vi "ALTS-2015 OPC Read Engine.vi"(8 "error in (no error)":errorcluster, 11 "Delay (ms)":u32=100) -> (0 "error out":errorcluster)   [LabVIEW 2013]
doc: "Copyright © 2005, Soliton Technologies.\nAll rights reserved."
uses:
  Controls/ALTS-2015 OPC Engine Main Options.ctl
  Controls/ALTS-2015 OPC Read Registers.ctl
  Controls/ALTS-2015 OPC Read Global Options.ctl
  Controls/ALTS-2015 OPC Global Options.ctl
  Controls/ALTS-2015 OPC Global Elements.ctl
  Globals/ALTS-2015 OPC Engine Globals.vi
  Controls/ALTS-2015 Safety Logic Cases.ctl
panel:
  in  "OPC Read Registers":T1=enum."Start_Test"
  out "Running Case":T2
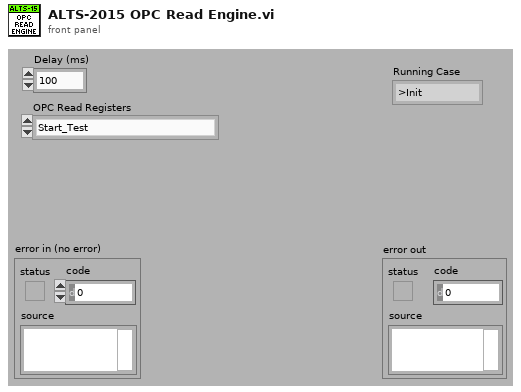
[diagram p1: front panel]
types:
  T1 = typedef "ALTS-2015 OPC Read Registers.ctl" = enum16{"Robot_Available", "Start_Test", "Stop_Test", "Scan_Trigger", "Station_No_Start_Stop_Test"}
  T2 = typedef "ALTS-2015 OPC Engine Main Options.ctl" = enum16{">Init", ">Safe Mode", ">Poll", ">Error", ">Exit", ">Write", ">Read", ">Restart"}
  T3 = typedef "ALTS-2015 OPC Global Options.ctl" = enum16{"Init", "Write 1", "Read 1", "Write Array", "Read Array", "Clear"}
  T4 = typedef "ALTS-2015 OPC Read Global Options.ctl" = enum16{"Init", "Write Value", "Write Array", "Read Value", "Read Array", "Read All"}
  T5 = cluster{"Channel Order":i32[], "Connection ids":refnum<k13>[]}
  T6 = enum16{"Read", "Write", "ReadWrite", "BufferedRead", "BufferedReadWrite"}
  T7 = typedef "ALTS-2015 OPC Global Elements.ctl" = enum16{"OPC - R Error", "OPC - W Error", "OPC - R Restart", "OPC - W Restart", "OPC - R Running", "OPC - W Running"}
  T8 = typedef "ALTS-2015 Safety Logic Cases.ctl" = enum16{"Read S/W EStop", "Read H/W EStop", "Write S/W EStop", "Write H/W EStop", "Read S/W & H/W EStop"}
  T9 = typedef "ALTS-2015 INI Configuration Cluster.ctl" = cluster{"Application":cluster{"Rerun Count":i32, "Workorder No":string}, "Station Details":cluster{"Sensor Name 1":string, "Sensor Name 2":string, "Sensor Name 3":string, "Sensor Name 4":string, "Station1 Enable":bool, "Station2 Enable":bool, "Station3 Enable":bool, "Station4 Enable":bool}, "Database":cluster{"Database Connection Link":path, "Result Procedure":string, "User":string, "Password":string, "Prompt":bool, "Station 1 LT Result DB DSN Path":path, "Station 2 LT Result DB DSN Path":path, "Station 3 LT Result DB DSN Path":path, "Station 4 LT Result DB DSN Path":path, "AirLeakTestResult Procedure":string, "Serial Details Procedure":string}, "Simulation":cluster{"Simulate DAQ Hardware":bool, "Simulate Result DB Write":bool, "Simulate Scanner":bool, "Simulate OPC":bool, "Simulate Serial Details DB":bool, "Simulate Result DB":bool, "Simulate Scanner DB Path":path, "Simulate Serial Details DB Path":path, "Simulate Result DB Path":path}, "Barcode Scanner1":cluster{"Scanner IP":string, "Scanner Port":u16, "#Bytes to Read":i32}, "Barcode Scanner2":cluster{"Enabled?":bool, "Scanner IP":string, "Scanner Port":u16, "#Bytes to Read":i32}}
  T10 = enum16{"Left Button", "Center Button", "Right Button", "Window Close"}
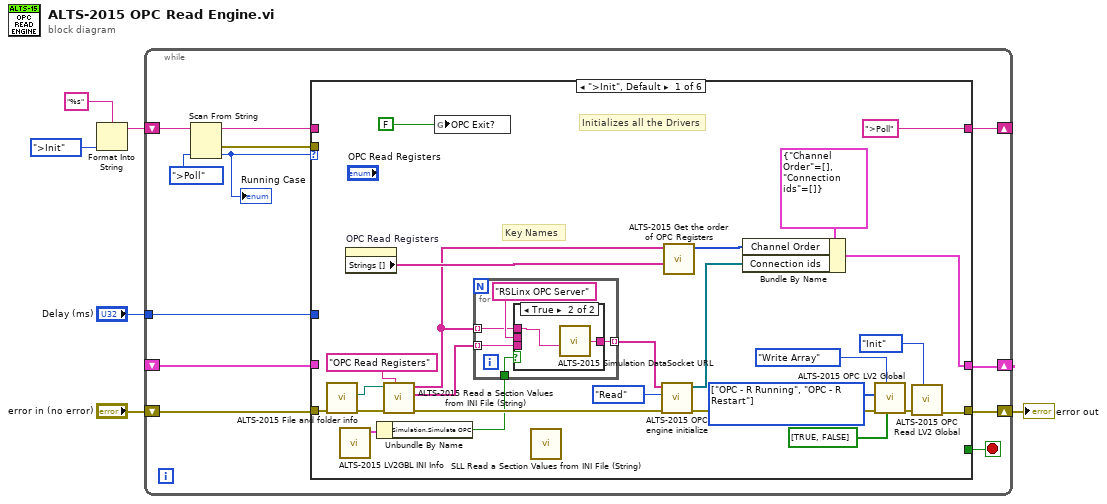
[diagram p0: block diagram]
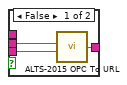
[diagram p2: hidden frame]
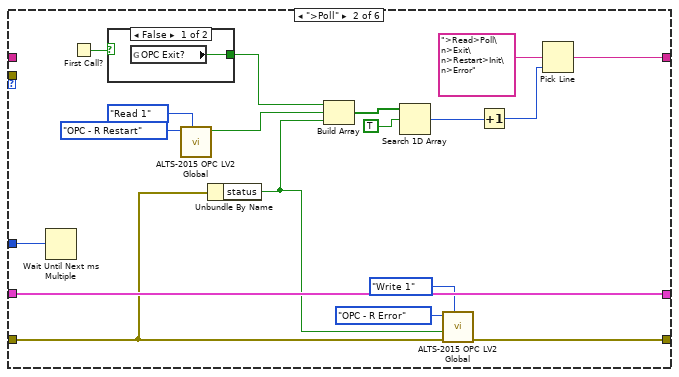
[diagram p3: hidden frame]
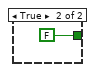
[diagram p4: hidden frame]
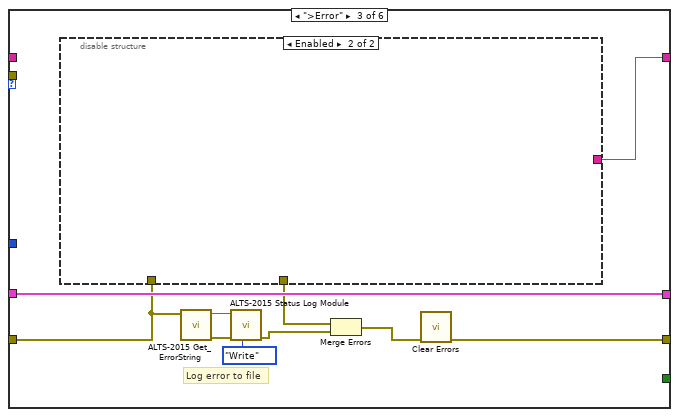
[diagram p5: hidden frame]
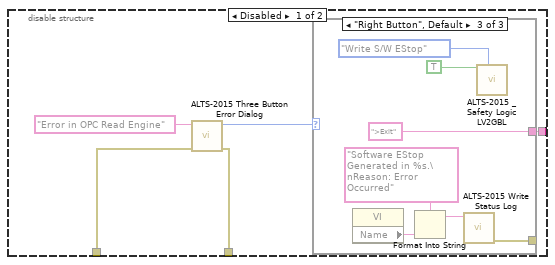
[diagram p6: hidden frame]
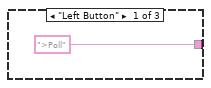
[diagram p7: hidden frame]
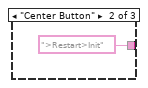
[diagram p8: hidden frame]
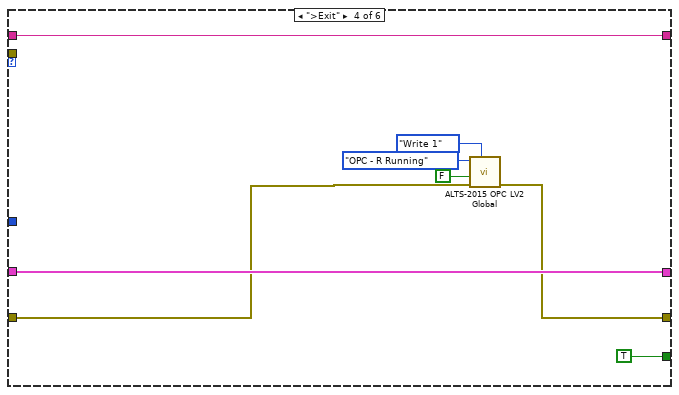
[diagram p9: hidden frame]
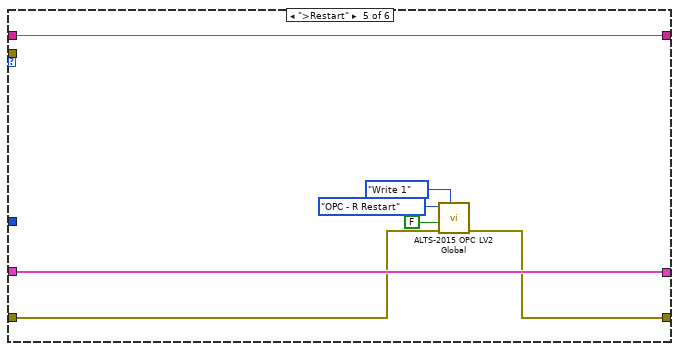
[diagram p10: hidden frame]
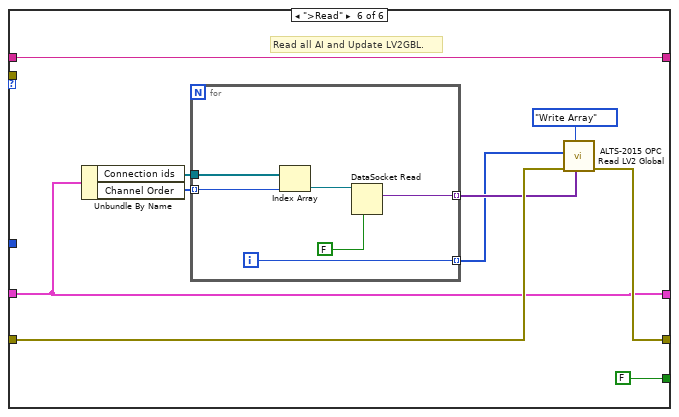
[diagram p11: hidden frame]
diagram:
  n1 = Format Into String(format string="%s", ALTS-2015_OPC_Engine_Main_Options.">Init" ("DAQ Options")) -> (resulting string=w2:string)  [unwired: 2 in, 1 out]
  n2 = while {
    shift-right: [w17] -> w5
    shift-left: "error in (no error)" -> [w18]
    shift-right: [w16] -> _
    shift-left: _ -> [w15]
    shift-right: [w10] -> _
    shift-left: w2 -> [w14]
    tunnel: "Delay (ms)" -> [w8]
    stop <- w9 stop-if-true
    n3 = Scan From String(input string=w14, default 1=ALTS-2015_OPC_Engine_Main_Options.">Poll" ("DAQ Options")) -> (remaining string=w12:string, error out=w11:errorcluster, output 1=w7:T2)  [unwired: 3 in, 1 out]
    "Running Case" <- w7
    n4 = case shown="\">Init\", Default" w7 {
      tunnel: w18 -> [w40 w60 w76 w98 w107 w119]
      tunnel: [w32 w59 w81 w99 w106 w120] -> w17
      tunnel: [w36 w71 w83 w105 w112 w113] -> w16
      tunnel: w15 -> [_ w71 w83 w105 w112 w113]
      tunnel: w12 -> [_ _ _ w104 w111 w122]
      tunnel: w11 -> [_ _ _ _ _ _]
      tunnel: [">Poll" ("output string") w65 w82 w104 w111 w122] -> w10
      tunnel: [_ _ _ TRUE _ FALSE] -> w9
      tunnel: w8 -> [_ w63 _ _ _ _]
      frame ">Init", Default {
        w25 = T7[] [enum."OPC - R Running", enum."OPC - R Restart"] items=["OPC - R Error", "OPC - W Error", "OPC - R Restart", "OPC - W Restart", "OPC - R Running", "OPC - W Running"] ("Elements Array")
        # "Key Names"
        # "Initializes all the Drivers"
        n5 = call "ALTS-2015 File and folder info.vi"("error in (no error)"=w40) -> ("error out"=w35:errorcluster, "INI file path"=w39:path)  [unwired: 2 in, 7 out]
        n6 = call "ALTS-2015 LV2GBL INI Info.vi"() -> ("Configuration Cluster Out"=w22:T9)  [unwired: 10 in, 1 out]
        n7 = property on="OPC Read Registers" class="Enum (strict)"() -> ("Strings []"=w34:string[])  [unwired: 2 in, 2 out]
        n8 = Unbundle By Name(w22) -> ("Simulation.Simulate OPC"=w23:bool)
        n9 = call "ALTS-2015 Read a Section Values from INI File (String).vi"("Section"="OPC Read Registers", "error in (no error)"=w35, "INI File Path"=w39) -> ("error out"=w42:errorcluster, "Key Values"=w21:string[], "Key Names"=w20:string[])  [unwired: 6 in]
        n10 = global write "ALTS-2015 OPC Engine Globals.vi" "OPC Exit?"(FALSE ("DAQ Exit?")) -> ()
        n11 = for {
          tunnel: w21 -> [w48] mode=indexing
          tunnel: [w47] -> w19 mode=indexing
          tunnel: w23 -> [w45]
          tunnel: w20 -> [w44] mode=indexing
          n12 = case shown="True" w45 {
            tunnel: w48 -> [w51 _]
            tunnel: [w50 w53] -> w47
            tunnel: "RSLinx OPC Server" ("Server Name") -> [w49 _]
            tunnel: w44 -> [_ w52]
            frame False {
              n13 = call "ALTS-2015 OPC To URL.vi"("Item Name"=w51, "Server Name"=w49) -> ("URL"=w50:string)  [unwired: 4 in]
            }
            frame True {
              n14 = call "ALTS-2015 Simulation DataSocket URL.vi"("Item Name"=w52) -> ("URL"=w53:string)  [unwired: 5 in]
            }
          }
        }
        n15 = call "SLL Read a Section Values from INI File (String).vi"() -> ()  [unwired: 8 in, 4 out]
        n16 = call "ALTS-2015 OPC engine initialize.vi"("error in (no error)"=w42, "mode"=T6."Read", "URLs"=w19) -> ("error out"=w27:errorcluster, "Connection ids"=w37:refnum<k13>[])  [unwired: 7 in]
        n17 = call "ALTS-2015 Get the order of OPC Registers.vi"("Register Names - Enum"=w34, "Register Names - INI"=w20) -> ("Channel Order"=w33:i32[])  [unwired: 8 in, 1 out]
        n18 = Bundle By Name(cluster=T5 {"Channel Order"=[], "Connection ids"=[]} ("Data Cluster"), "Channel Order"=w33, "Connection ids"=w37) -> (w36:T5)
        n19 = call "ALTS-2015 OPC LV2 Global.vi"("Status Array In"=bool[] [TRUE, FALSE], "Option"=ALTS-2015_OPC_Global_Options."Write Array", "error in (no error)"=w27, "Elements Array"=w25) -> ("error out"=w26:errorcluster)  [unwired: 5 in, 2 out]
        n20 = call "ALTS-2015 OPC Read LV2 Global.vi"("Options"=ALTS-2015_OPC_Read_Global_Options."Init", "error in (no error)"=w26) -> ("error out"=w32:errorcluster)  [unwired: 7 in, 2 out]
      }
      frame ">Poll" {
        n21 = Wait Until Next ms Multiple(millisecond multiple=w63) -> ()  [unwired: 1 out]
        n22 = First Call?() -> (First Call?: T/F=w55:bool)
        n23 = case shown="False" w55 {
          tunnel: [w72 FALSE ("OPC Exit?")] -> w64
          frame False {
            n24 = global read "ALTS-2015 OPC Engine Globals.vi" "OPC Exit?"() -> (w72:bool)
          }
          frame True {
          }
        }
        n25 = call "ALTS-2015 OPC LV2 Global.vi"("Option"=ALTS-2015_OPC_Global_Options."Read 1", "Elements"=ALTS-2015_OPC_Global_Elements."OPC - R Restart") -> ("Status Out"=w62:bool)  [unwired: 7 in, 2 out]
        n26 = Unbundle By Name(w60) -> ("status"=w58:bool)
        n27 = Build Array(w64, w62, w58) -> (w69:bool[])
        n28 = Search 1D Array(1D array=w69, element=TRUE) -> (index of element=w67:i32)  [unwired: 1 in]
        n29 = call "ALTS-2015 OPC LV2 Global.vi"("Option"=ALTS-2015_OPC_Global_Options."Write 1", "error in (no error)"=w60, "Status In"=w58, "Elements"=ALTS-2015_OPC_Global_Elements."OPC - R Error") -> ("error out"=w59:errorcluster)  [unwired: 5 in, 2 out]
        n30 = Increment(x=w67) -> (x+1=w66:i32)
        n31 = Pick Line(multi-line string=">Read>Poll\n>Exit\n>Restart>Init\n>Error", line index=w66) -> (output string=w65:string)  [unwired: 1 in]
      }
      frame ">Error" {
        # "Log error to file"
        n32 = disable-structure shown="Enabled" {
          disable-tunnel: [w86 _] -> w82
          disable-tunnel: w76 -> [w85 _]
          disable-tunnel: [w84 _] -> w75
          frame Disabled {
            n33 = call "ALTS-2015 Three Button Error Dialog.vi"("Error In"=w85, "Window Title"="Error in OPC Read Engine") -> ("Error Out"=w84:errorcluster, "Which Button?"=w87:T10)  [unwired: 8 in]
            n34 = case shown="\"Right Button\", Default" w87 {
              tunnel: [">Poll" ("format string") ">Restart>Init" ("format string") ">Exit" ("format string")] -> w86
              tunnel: [_ _ w91] -> _
              frame "Left Button" {
              }
              frame "Center Button" {
              }
              frame "Right Button", Default {
                n35 = property class="VI"() -> ("Name"=w93:string)  [unwired: 2 in, 2 out]
                n36 = Format Into String(format string="Software EStop Generated in %s.\nReason: Error Occurred" ("Status Input"), w93) -> (resulting string=w94:string)  [unwired: 2 in, 1 out]
                n37 = call "ALTS-2015 Write Status Log.vi"("Status Input"=w94) -> ("error out"=w91:errorcluster)  [unwired: 10 in]
                n38 = call "ALTS-2015 _Safety Logic LV2GBL.vi"("Options"=ALTS-2015_Safety_Logic_Cases."Write S/W EStop", "EStop In"=TRUE) -> ()  [unwired: 6 in, 4 out]
              }
            }
          }
          frame Enabled {
          }
        }
        n39 = call "ALTS-2015 Get_ErrorString.vi"("Incoming Error"=w76) -> ("error out"=w77:errorcluster, "Message"=w79:string)  [unwired: 9 in]
        n40 = call "ALTS-2015 Status Log Module.vi"("Options"=enum16{"Init", "Write", "Close"}."Write", "error in"=w77, "Text to  Log"=w79) -> ("error out"=w78:errorcluster)  [unwired: 8 in]
        n41 = Merge Errors(w75, w78) -> (w74:errorcluster)
        n42 = call <vilib>:"Clear Errors.vi"("error in (no error)"=w74) -> ("error out"=w81:errorcluster)  [unwired: 6 in]
      }
      frame ">Exit" {
        n43 = call "ALTS-2015 OPC LV2 Global.vi"("Option"=ALTS-2015_OPC_Global_Options."Write 1", "error in (no error)"=w98, "Status In"=FALSE, "Elements"=ALTS-2015_OPC_Global_Elements."OPC - R Running") -> ("error out"=w99:errorcluster)  [unwired: 5 in, 2 out]
      }
      frame ">Restart" {
        n44 = call "ALTS-2015 OPC LV2 Global.vi"("Option"=ALTS-2015_OPC_Global_Options."Write 1", "error in (no error)"=w107, "Status In"=FALSE, "Elements"=ALTS-2015_OPC_Global_Elements."OPC - R Restart") -> ("error out"=w106:errorcluster)  [unwired: 5 in, 2 out]
      }
      frame ">Read" {
        # "Read all AI and Update LV2GBL."
        n45 = Unbundle By Name(w113) -> ("Connection ids"=w116:refnum<k13>[], "Channel Order"=w117:i32[])
        n46 = for {
          tunnel: [w128] -> w115 mode=indexing
          tunnel: w117 -> [w126] mode=indexing
          tunnel: w116 -> [w127]
          tunnel: [w123] -> w114 mode=indexing
          i -> [w123]
          n47 = Index Array(array=w127, index=w126) -> (element=w125:refnum<k13>)
          n48 = DataSocket Read(6:FALSE ("wait for updated value (T)"), 11:w125) -> (2:w128:variant)  [unwired: 3 in, 6 out]
        }
        n49 = call "ALTS-2015 OPC Read LV2 Global.vi"("OPC value Array"=w115, "Options"=ALTS-2015_OPC_Read_Global_Options."Write Array", "error in (no error)"=w119, "OPC Read Register Array"=w114) -> ("error out"=w120:errorcluster)  [unwired: 5 in, 2 out]
      }
    }
  }
  "error out" <- w5
